vi "App_Search Data.vi"(8 "error in":errorcluster) -> (0 "error out":errorcluster, 3 "Log Data":T1[](array[typedef]))   [LabVIEW 2015, in "Application 2.lvlib"]
uses:
  Application 2.lvlib
  Com VIs/Data Def/Data File Format.ctl
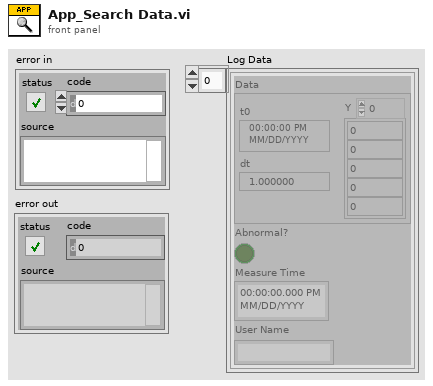
[diagram p1: front panel]
types:
  T1 = typedef "Data File Format.ctl" = cluster{"Data":waveform(dbl), "Abnormal?":bool, "Measure Time":timestamp, "User Name":string}
  T2 = typedef "Application 2.lvlib/App_Main Data.ctl" = cluster{"VI Refnum":refnum<vi>, "Subpanel":refnum<vi>, "Connection ID":refnum<k5>, "Meta data":T3[], "Main Queue":T5, "User Data":T6}
  T3 = typedef "stm_MetaElement.ctl" = cluster{"Name":T4}
  T4 = typedef "stm_MetaDataElement.ctl" = string
  T5 = typedef "Application 2.lvlib/App_Main Queue.ctl" = cluster{"Main Loop Queue":refnum<queue>}
  T6 = typedef "User Data.ctl" = cluster{"Name":string, "Email":string, "Phone Number":string, "User Picture":u32[][], "Last Login Time":timestamp}
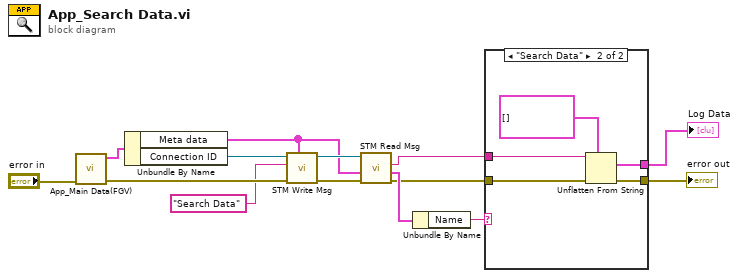
[diagram p0: block diagram]
diagram:
  n1 = call "App_Main Data(FGV).vi"("error in"="error in") -> ("error out"=w11:errorcluster, "Main Data Out"=w13:T2)  [unwired: 9 in]
  n2 = Unbundle By Name(w13) -> ("Meta data"=w7:T3[], "Connection ID"=w12:refnum<k5>)
  n3 = call "STM Write Msg.vi"("Meta data"=w7, "error in (no error)"=w11, "Name"="Search Data", "connection ID"=w12) -> ("error out"=w9:errorcluster, "connection ID out"=w8:refnum<k5>)  [unwired: 6 in]
  n4 = call "STM Read Msg.vi"("error in"=w9, "Meta data"=w7, "connection ID"=w8) -> ("error out"=w4:errorcluster, "Meta element"=w6:T3, "data string"=w3:string)  [unwired: 3 in, 3 out]
  n5 = Unbundle By Name(w6) -> ("Name"=w5:T4)
  n6 = case shown="\"Search Data\"" w5 {
    tunnel: w4 -> [w15 w20]
    tunnel: w3 -> [_ w19]
    tunnel: [_ w17] -> w2
    tunnel: [w15 w16] -> w1
    frame Default {
    }
    frame "Search Data" {
      n7 = Unflatten From String(type=T1[] [] ("Array"), binary string=w19, error in (no error)=w20) -> (value=w17:T1[], error out=w16:errorcluster)  [unwired: 2 in, 1 out]
    }
  }
  "error out" <- w1
  "Log Data" <- w2
